vi "phy_symbol_gen.vi"(8 "type":enum16{"binary", "quadrature"}(ring), 11 "Input bytes":u8[](array[numeric])) -> (3 "symbols":cdb[](array[numeric]))   [LabVIEW 2014]
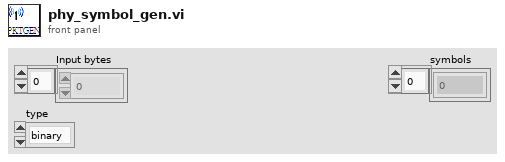
[diagram p1: front panel]
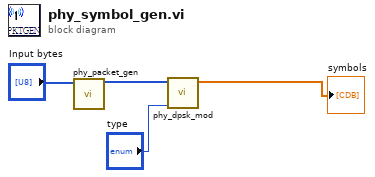
[diagram p0: block diagram]
diagram:
  n1 = call "phy_packet_gen.vi"("Input bytes"="Input bytes") -> ("output bit stream"=w4:i8[])  [unwired: 10 in]
  n2 = call "phy_dpsk_mod.vi"("type"="type", "input bits"=w4) -> ("dpsk"=→"symbols":cdb[])  [unwired: 8 in, 1 out]
